vi "Calc_Xray_travel_from_Z_travel.vi"(6 "Z tilt (degrees)":dbl, 11 "Z travel (steps)":dbl) -> (1 "X-ray travel (steps)":i32, 3 "Z travel (steps)":i32)   [LabVIEW 2018]
uses:
  ConversionAndInformation/Unit_Control.ctl
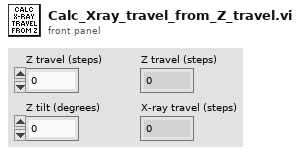
[diagram p1: front panel]
types:
  T1 = typedef "Unit_Control.ctl" = enum16{"Angle (Degrees)", "Rad", "Angle [TMC]", "Microsteps [TMC]", "Inches", "Nanometer", "Meter", "Centimeter", "Millimeter", "Micron"}
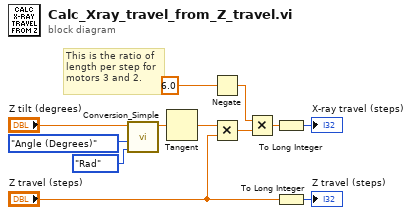
[diagram p0: block diagram]
diagram:
  # "This is the ratio of\nlength per step for\nmotors 3 and 2."
  n1 = call "Conversion_Simple.vi"("Output Unit"=Unit_Control."Rad", "Input Unit"=Unit_Control."Angle (Degrees)", "Input"="Z tilt (degrees)") -> ("Output"=w11:dbl)  [unwired: 7 in, 1 out]
  n2 = Tangent(1:w11) -> (0:w10:dbl)
  n3 = Negate(x=6.0) -> (-x=w2:dbl)
  n4 = Multiply(x=w10, y="Z travel (steps)") -> (x*y=w9:dbl)
  n5 = Multiply(x=w2, y=w9) -> (x*y=w8:dbl)
  n6 = To Long Integer(number=w8) -> (32bit integer=→"X-ray travel (steps)":i32)
  n7 = To Long Integer(number="Z travel (steps)") -> (32bit integer=→"Z travel (steps)":i32)
